vi "iTCset.vi"(8 "error in (no error)":errorcluster, 9 "Set Point":dbl min=0.0 max=100.0 step=0.01, 10 "iTCSetCtrl":T1, 11 "VISA resource name":refnum<visa-resource-name>) -> (0 "error out":errorcluster, 1 "read buffer":string, 2 "number":dbl, 3 "VISA resource name out":refnum<visa-resource-name>)   [LabVIEW 2021]
uses:
  controls/iTCsetCtrl.ctl
  <vilib>/regexp/Match Regular Expression.xnode
panel:
  in  "Set":bool
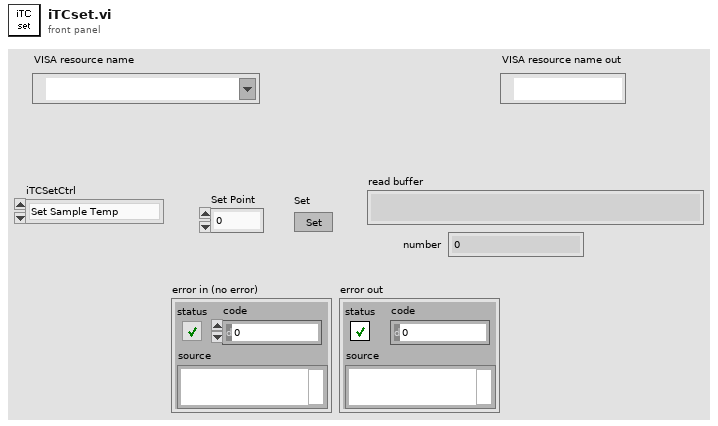
[diagram p1: front panel]
types:
  T1 = typedef "iTCsetCtrl.ctl" = enum16{"Set Sample Temp", "Set VTI Temp", "Set Needle Valve", "Set VTI Heater Power", "Set Sample Heater Power", "Set VTI Pressure"}
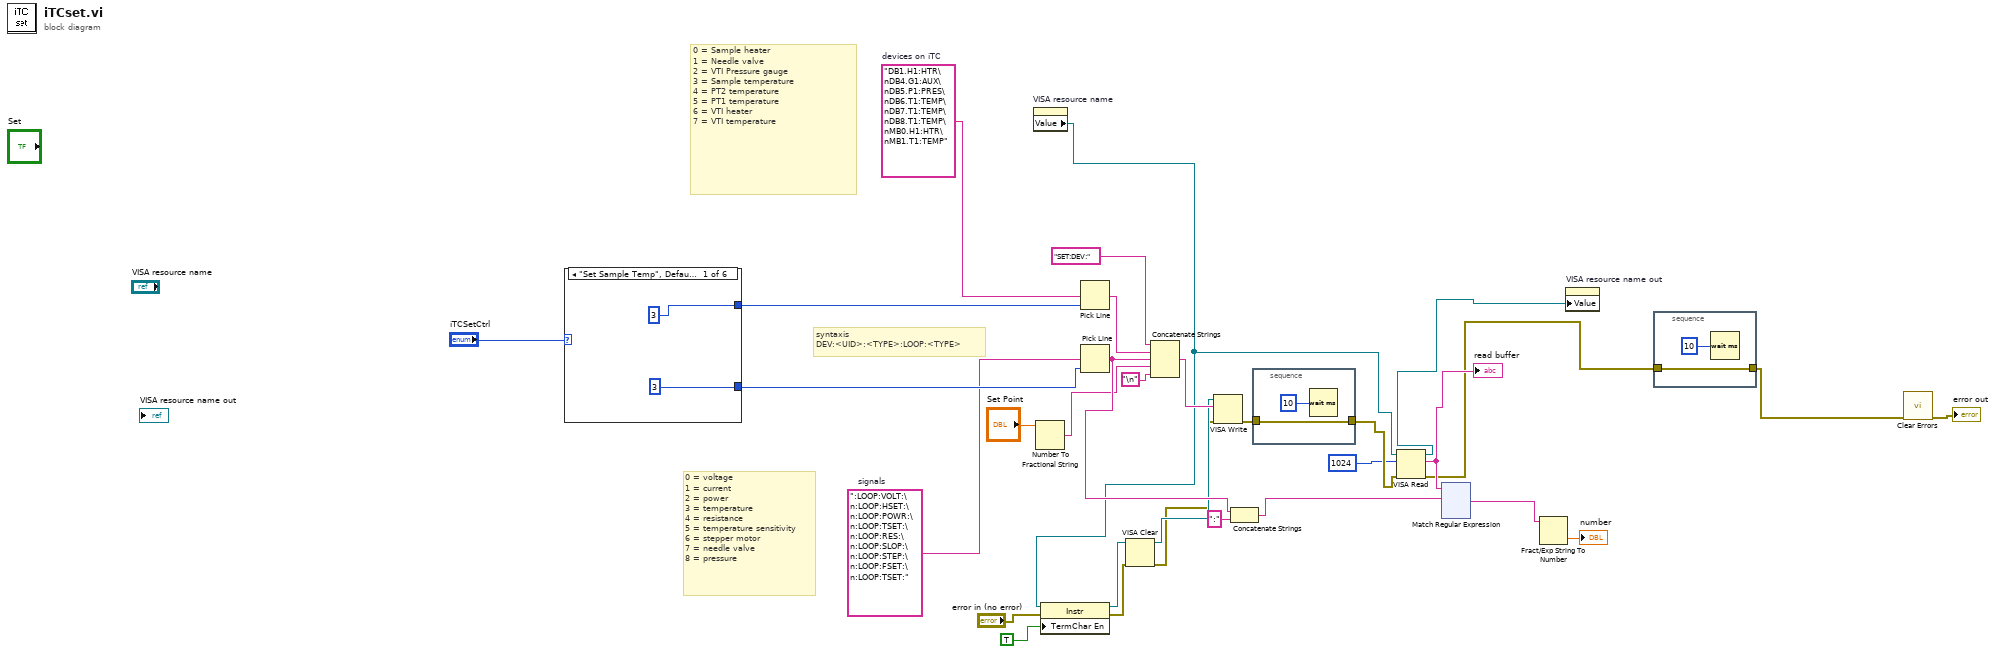
[diagram p0: block diagram]
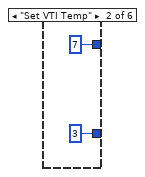
[diagram p2: hidden frame]
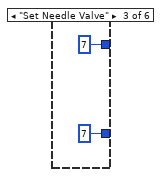
[diagram p3: hidden frame]
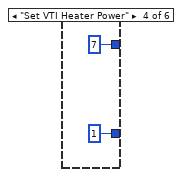
[diagram p4: hidden frame]
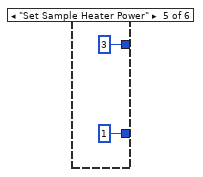
[diagram p5: hidden frame]
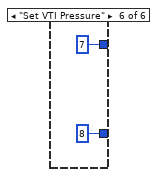
[diagram p6: hidden frame]
diagram:
  w17 = ":LOOP:VOLT:\n:LOOP:HSET:\n:LOOP:POWR:\n:LOOP:TSET:\n:LOOP:RES:\n:LOOP:SLOP:\n:LOOP:STEP:\n:LOOP:FSET:\n:LOOP:TSET:"  # signals
  w15 = "DB1.H1:HTR\nDB4.G1:AUX\nDB5.P1:PRES\nDB6.T1:TEMP\nDB7.T1:TEMP\nDB8.T1:TEMP\nMB0.H1:HTR\nMB1.T1:TEMP"  # devices on iTC
  # "0 = Sample heater\n1 = Needle valve\n2 = VTI Pressure gauge\n3 = Sample temperature\n4 = PT2 temperature\n5 = PT1 temperature\n6 = VTI heater\n7 = VTI temperature"
  # "0 = voltage\n1 = current\n2 = power\n3 = temperature\n4 = resistance\n5 = temperature sensitivity\n6 = stepper motor\n7 = needle valve\n8 = pressure"
  # "syntaxis\nDEV:<UID>:<TYPE>:LOOP:<TYPE>"
  n1 = case shown="\"Set Sample Temp\", Default" "iTCSetCtrl" {
    tunnel: [3 ("line index") 7 ("line index") 7 ("line index") 7 ("line index") 3 ("line index") 7 ("line index")] -> w25
    tunnel: [3 ("line index") 3 ("line index") 7 ("line index") 1 ("line index") 1 ("line index") 8 ("line index")] -> w26
    frame "Set Sample Temp", Default {
    }
    frame "Set VTI Temp" {
    }
    frame "Set Needle Valve" {
    }
    frame "Set VTI Heater Power" {
    }
    frame "Set Sample Heater Power" {
    }
    frame "Set VTI Pressure" {
    }
  }
  n2 = property on="VISA resource name" class="VISAName"() -> ("Value"=w7:refnum<visa-resource-name>)  [unwired: 2 in, 2 out]
  n3 = Number To Fractional String(number="Set Point") -> (F-format string=w12:string)  [unwired: 3 in]
  n4 = property class="Instr"(reference=w7, error in="error in (no error)", "TermChar En"=TRUE ("Message Based Settings:Termination Character Enable")) -> (reference out=w6:refnum<visa-resource-name>, error out=w5:errorcluster)
  n5 = Pick Line(multi-line string=w15, line index=w25) -> (output string=w21:string)  [unwired: 1 in]
  n6 = Pick Line(multi-line string=w17, line index=w26) -> (output string=w23:string)  [unwired: 1 in]
  n7 = VISA Clear(VISA resource name=w6, error in (no error)=w5) -> (VISA resource name out=w8:refnum<visa-resource-name>, error out=w4:errorcluster)
  n8 = Concatenate Strings("SET:DEV:" ("write buffer"), w21, w23, w12, "\n") -> (w22:string)
  n9 = VISA Write(VISA resource name=w8, write buffer=w22, error in (no error)=w4) -> (error out=w20:errorcluster)  [unwired: 2 out]
  n10 = Concatenate Strings(w23, ":" ("string")) -> (w24:string)
  n11 = stacked-sequence {
    tunnel: w20 -> [w45]
    tunnel: [w45] -> w29
    frame #0 {
      n12 = Wait (ms)(milliseconds to wait=u32 10) -> ()  [unwired: 1 out]
    }
  }
  n13 = VISA Read(VISA resource name=w7, byte count=u32 1024, error in (no error)=w29) -> (VISA resource name out=w1:refnum<visa-resource-name>, read buffer=w30:string, error out=w2:errorcluster)  [unwired: 1 out]
  "read buffer" <- w30
  n14 = xnode "Match Regular Expression"("input string"=w30, "regular expression"=w24) -> ("after match"=w27:string)  [unwired: 4 in, 4 out]
  n15 = Fract/Exp String To Number(string=w27) -> (number=→"number":dbl)  [unwired: 3 in, 1 out]
  n16 = property on="VISA resource name out" class="VISAName"("Value"=w1) -> ()  [unwired: 2 in, 2 out]
  n17 = stacked-sequence {
    tunnel: w2 -> [w46]
    tunnel: [w46] -> w3
    frame #0 {
      n18 = Wait (ms)(milliseconds to wait=u32 10) -> ()  [unwired: 1 out]
    }
  }
  n19 = call <vilib>:"Clear Errors.vi"("error in (no error)"=w3) -> ("error out"=→"error out":errorcluster)  [unwired: 5 in, 1 out]
